vi "Autosort Initialise.vi"(8 "error in (no error)":errorcluster) -> (0 "error out":errorcluster)   [LabVIEW 2016]
uses:
  Autosort Parameters.ctl
  Autosort Parameters Set.vi
panel:
  in  "Default Autosort Parameters":T1={"Name"="Default", "Min Vel"=20.0, "Trigger Ch"=1, "MaxVel"=300.0, "Width"=100, "Pre Impuls"=150, "Post Impuls"=150, "Pitch"=15.0, "Other Trigger"=FALSE, "Cross Corr"=FALSE}
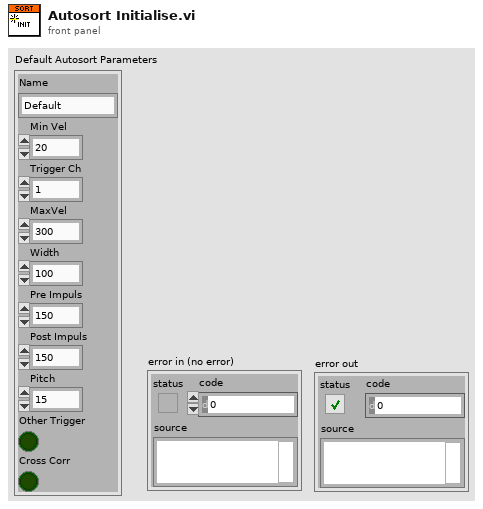
[diagram p1: front panel]
types:
  T1 = typedef "Autosort Parameters.ctl" = cluster{"Name":string, "Min Vel":dbl, "Trigger Ch":i32, "MaxVel":dbl, "Width":i32, "Pre Impuls":i32, "Post Impuls":i32, "Pitch":dbl, "Other Trigger":bool, "Cross Corr":bool}
  T2 = enum16{"open", "replace", "create", "open or create", "replace or create", "replace or create with confirmation"}
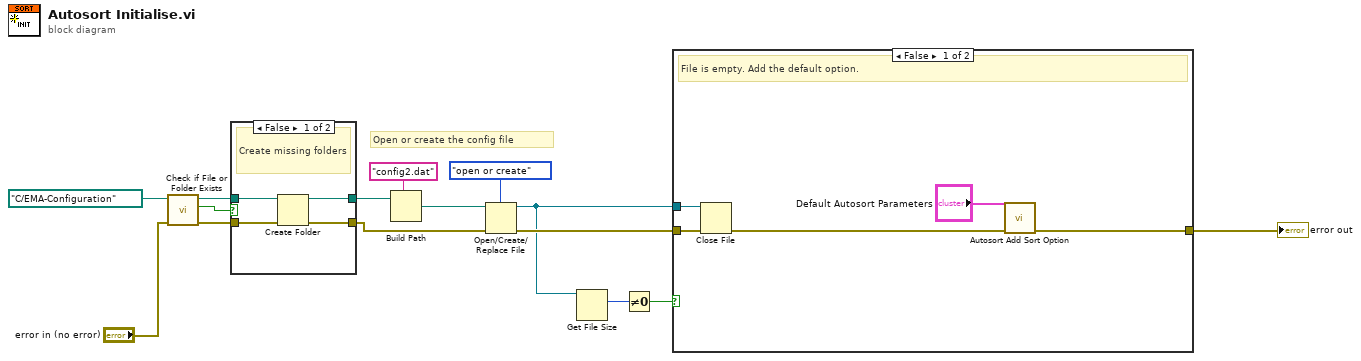
[diagram p0: block diagram]
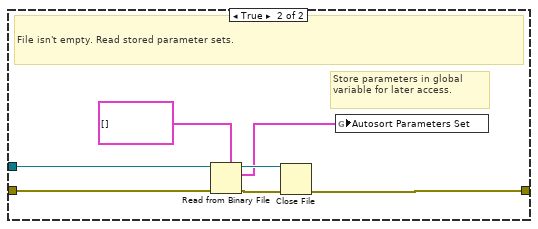
[diagram p2: hidden frame]
diagram:
  # "Open or create the config file"
  n1 = call <vilib>:"Check if File or Folder Exists.vi"("error in (no error)"="error in (no error)", "path"=path "C:/EMA-Configuration") -> ("error out"=w13:errorcluster, "file or folder exists?"=w11:bool, "dup path"=w12:path)  [unwired: 7 in]
  n2 = case shown="False" w11 {
    tunnel: w13 -> [w19 w20]
    tunnel: w12 -> [w18 w21]
    tunnel: [w16 w21] -> w10
    tunnel: [w17 w20] -> w7
    frame False {
      # "Create missing folders"
      n3 = Create Folder(path (use dialog)=w18, error in=w19) -> (created path=w16:path, error out=w17:errorcluster)  [unwired: 1 in, 1 out]
    }
    frame True {
    }
  }
  n4 = Build Path(base path=w10, name or relative path="config2.dat") -> (appended path=w1:path)
  n5 = Open/Create/Replace File(file path (use dialog)=w1, error in=w7, operation (0:open)=T2."open or create") -> (refnum out=w5:refnum<file>, error out=w6:errorcluster)  [unwired: 3 in, 1 out]
  n6 = Get File Size(file=w5) -> (size (in bytes)=w4:i64)  [unwired: 1 in, 2 out]
  n7 = Not Equal To 0?(x=w4) -> (x != 0?=w3:bool)
  n8 = case shown="False" w3 {
    tunnel: w6 -> [w25 w33]
    tunnel: w5 -> [w26 w32]
    tunnel: [w22 w29] -> w2
    frame False {
      # "File is empty. Add the default option."
      n9 = Close File(refnum=w26, error in=w25) -> (error out=w24:errorcluster)  [unwired: 1 out]
      n10 = call "Autosort Add Sort Option.vi"("error in (no error)"=w24, "Autosort Parameters"="Default Autosort Parameters") -> ("error out"=w22:errorcluster)  [unwired: 8 in, 1 out]
    }
    frame True {
      # "Store parameters in global variable for later access."
      # "File isn't empty. Read stored parameter sets."
      n11 = Read from Binary File(5:T1[] [] ("Array"), 8:w33, 11:w32) -> (0:w30:errorcluster, 2:w28:T1[], 3:w31:refnum<file>)  [unwired: 3 in, 1 out]
      n12 = Close File(refnum=w31, error in=w30) -> (error out=w29:errorcluster)  [unwired: 1 out]
      n13 = global write "Autosort Parameters Set.vi" "Autosort Parameters Set"(w28) -> ()
    }
  }
  "error out" <- w2
